vi "BackgroundHWT.vi"(1 "Sample Time(seconds)":dbl=50.0 format="%0.2f") -> (0 "Counts":i32)   [LabVIEW 2012]
uses:
  <vilib>/DAQmx/read.llb/DAQmx Read (Counter U32 1Chan 1Samp).vi
  <vilib>/DAQmx/create/channels.llb/DAQmx Create Channel (CO-Pulse Generation-Frequency).vi
  <vilib>/DAQmx/configure/timing.llb/DAQmx Timing (Implicit).vi
  <vilib>/DAQmx/create/channels.llb/DAQmx Create Channel (CI-Count Edges).vi
  <vilib>/DAQmx/configure/timing.llb/DAQmx Timing (Sample Clock).vi
  <vilib>/DAQmx/miscellaneous.llb/DAQmx Fill In Error Info.vi
  <resource>/objmgr/daqmx.rc
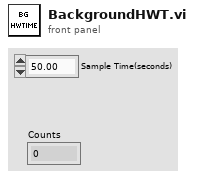
[diagram p1: front panel]
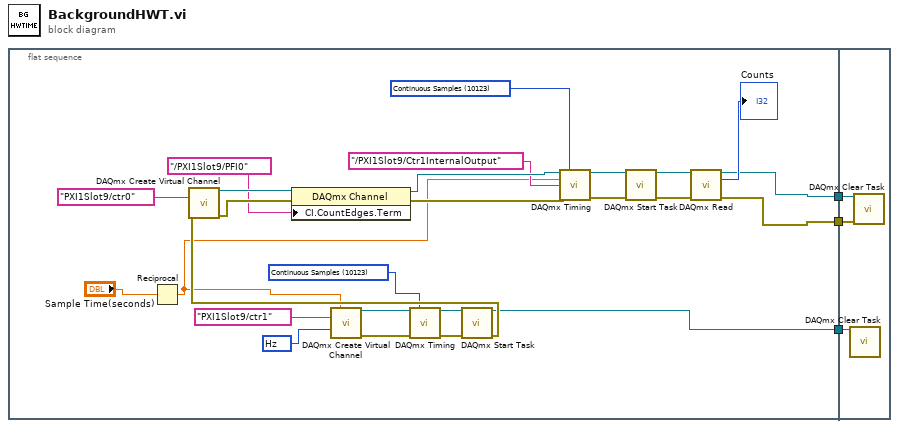
[diagram p0: block diagram]
diagram:
  n1 = flat-sequence {
    tunnel: [w6] -> w3
    tunnel: [w5] -> w2
    tunnel: [w4] -> w1
    tunnel: w3 -> [w32]
    tunnel: w2 -> [w31]
    tunnel: w1 -> [w30]
    frame #0 {
      w12 = 10123 items=["Finite Samples"=10178, "Continuous Samples"=10123, "Hardware Timed Single Point"=12522] ("sample mode")
      w18 = 10373 items=["Hz"=10373] ("units")
      w21 = 10123 items=["Finite Samples"=10178, "Continuous Samples"=10123, "Hardware Timed Single Point"=12522] ("sample mode")
      n2 = Reciprocal(x="Sample Time(seconds)") -> (1/x=w8:dbl)
      n3 = call-poly <vilib>:"DAQmx Create Virtual Channel.vi"("frequency"=w8, "counter"=tag "PXI1Slot9/ctr1", "units"=w18) -> ("task out"=w16:refnum<k21>, "error out"=w15:errorcluster)  [unwired: 11 in]
      n4 = call-poly <vilib>:"DAQmx Timing.vi"("task/channels in"=w16, "sample mode"=w12, "error in"=w15) -> ("task out"=w14:refnum<k21>, "error out"=w13:errorcluster)  [unwired: 11 in]
      n5 = call <vilib>:"DAQmx Start Task.vi"("task/channels in"=w14, "error in"=w13) -> ("task out"=w4:refnum<k21>, "error out"=w19:errorcluster)  [unwired: 12 in]
      n6 = call-poly <vilib>:"DAQmx Create Virtual Channel.vi"("counter"=tag "PXI1Slot9/ctr0", "error in"=w19) -> ("task out"=w24:refnum<k21>, "error out"=w23:errorcluster)  [unwired: 12 in]
      n7 = property class="DAQmx Channel"(reference=w24, error in=w23, "CI.CountEdges.Term"=tag "/PXI1Slot9/PFI0") -> (reference out=w26:refnum<k21>, error out=w25:errorcluster)
      n8 = call-poly <vilib>:"DAQmx Timing.vi"("task/channels in"=w26, "sample mode"=w21, "rate"=w8, "source"=tag "/PXI1Slot9/Ctr1InternalOutput", "error in"=w25) -> ("task out"=w28:refnum<k21>, "error out"=w27:errorcluster)  [unwired: 9 in]
      n9 = call <vilib>:"DAQmx Start Task.vi"("task/channels in"=w28, "error in"=w27) -> ("task out"=w11:refnum<k21>, "error out"=w10:errorcluster)  [unwired: 12 in]
      n10 = call-poly <vilib>:"DAQmx Read.vi"("task/channels in"=w11, "error in"=w10) -> ("task out"=w6:refnum<k21>, "data"=→"Counts":u32, "error out"=w5:errorcluster)  [unwired: 11 in]
    }
    frame #1 {
      n11 = call <vilib>:"DAQmx Clear Task.vi"("task in"=w30) -> ()  [unwired: 14 in, 1 out]
      n12 = call <vilib>:"DAQmx Clear Task.vi"("task in"=w32, "error in"=w31) -> ()  [unwired: 13 in, 1 out]
    }
  }
